vi "Set FixedRows.vi"(8 "error in (no error)":errorcluster, 10 "FixedRows":i32, 11 "Sourcegrid in":refnum<class "SourceGrid.lvclass">) -> (0 "error out":errorcluster, 3 "Sourcegrid out":refnum<class "SourceGrid.lvclass">)   [LabVIEW 2024, in "SourceGrid.lvlib" / "SourceGrid.lvclass"]
uses:
  SourceGrid.lvclass
  SourceGrid.lvclass/SourceGrid.ctl
  D:/git/Sourcegrid-LabVIEW/dll/SourceGrid.dll
  dll/SourceGrid.dll
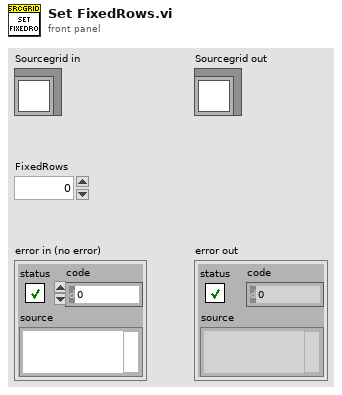
[diagram p1: front panel]
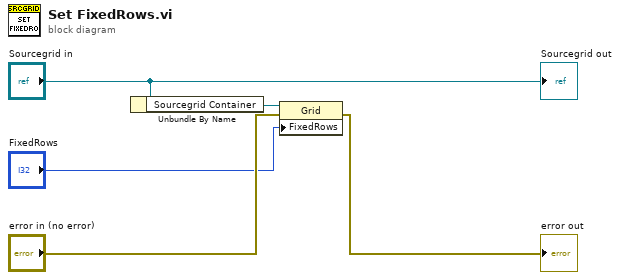
[diagram p0: block diagram]
diagram:
  n1 = Unbundle By Name("Sourcegrid in") -> ("Sourcegrid Container"=w1:refnum<k24>)
  n2 = property class="Grid"(reference=w1, error in="error in (no error)", "FixedRows"="FixedRows") -> (error out=→"error out":errorcluster)  [unwired: 1 out]
  "Sourcegrid out" <- "Sourcegrid in"
